vi "Allocate Millisecond Tick Timers.vi"(8 "error in (no error)":errorcluster, 10 "QtyTimers":i32, 11 "DbgTimers in":refnum<class "DbgTimers.lvclass">) -> (0 "error out":errorcluster, 3 "DbgTimers out":refnum<class "DbgTimers.lvclass">)   [LabVIEW 2017, in "DbgTimers.lvclass"]
doc: "Developed by Kevin Thompson\nkevin@thompsonengineering.net\n\nCopyright 2018-2020\nThompson Engineering, LLC"
uses:
  DbgTimers.lvclass
  DataTypes/Millisecond Tick Timer--cluster.ctl
  DbgTimers.lvclass/DbgTimers.ctl
  Accessors/Get ObjData.vi
  Accessors/Set ObjData.vi
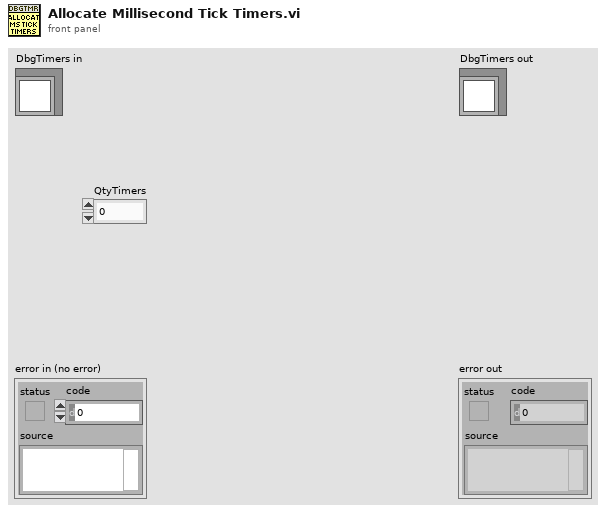
[diagram p1: front panel]
types:
  T1 = typedef "DbgTimers.lvclass/Millisecond Tick Timer--cluster.ctl" = cluster{"startTick":u32, "currentTick":u32, "elapsedTicks":u32, "totalElapsedTicks":u32}
  T2 = typedef "DbgTimers.lvclass/ObjData--cluster.ctl" = cluster{"Settings":T3, "ReadData-placeholder":T4, "Timers":T5, "Enable msTick Logging":bool, "LogFile_msTickTimer":path}
  T3 = typedef "DbgTimers.lvclass/Settings--cluster.ctl" = cluster{"Simulation":bool, "DbgTimer LogFolder":path}
  T4 = typedef "DbgTimers.lvclass/Read Data--cluster.ctl" = cluster{"Data":dbl}
  T5 = typedef "DbgTimers.lvclass/Timers--cluster.ctl" = cluster{"ms tick timers":T1[]}
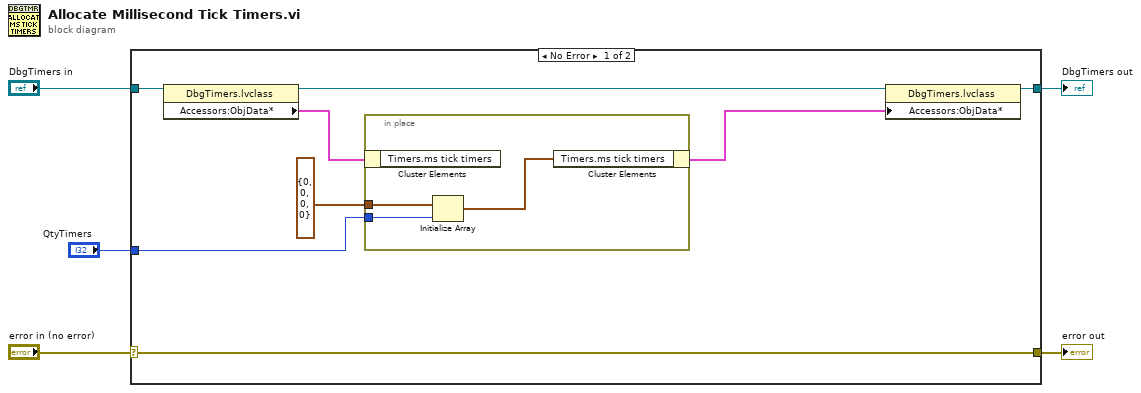
[diagram p0: block diagram]
diagram:
  n1 = case shown="No Error" "error in (no error)" {
    selector: "error in (no error)" -> [w12 w18]
    tunnel: [w12 w18] -> w4
    tunnel: [w10 w17] -> w2
    tunnel: "DbgTimers in" -> [w13 w17]
    tunnel: "QtyTimers" -> [w7 _]
    frame No Error {
      n2 = property class="DbgTimers.lvclass"(reference=w13) -> (reference out=w11:refnum<class "DbgTimers.lvclass">, "Accessors:ObjData*"=w9:T2)  [unwired: 1 in, 1 out]
      n3 = in-place {
        in-place-border: T1 {"startTick"=0, "currentTick"=0, "elapsedTicks"=0, "totalElapsedTicks"=0} ("ms tick timer") -> [w16]
        in-place-border: w7 -> [w15]
        n4 = in-place-cluster #1(w9) -> ()  [unwired: 1 out]
        n5 = Initialize Array(w16, w15) -> (w14:T1[])
        n6 = in-place-cluster #1("Timers.ms tick timers"=w14) -> (w6:T2)
      }
      n7 = property class="DbgTimers.lvclass"(reference=w11, "Accessors:ObjData*"=w6) -> (reference out=w10:refnum<class "DbgTimers.lvclass">)  [unwired: 1 in, 1 out]
    }
    frame Error {
    }
  }
  "error out" <- w4
  "DbgTimers out" <- w2
